vi "Progress Bar Example.vi"() -> ()   [LabVIEW 2015]
uses:
  <vilib>/Utility/sysdir.llb/System Directory Type.ctl
  Library/New Job Status.vi
  Library/New Item Status.vi
  Library/New Item Progression.vi
  Library/Finish.vi
  Library/Simple Progress Bar.lvlib
panel:
  out "Waiting for User":bool
  out "error out":errorcluster
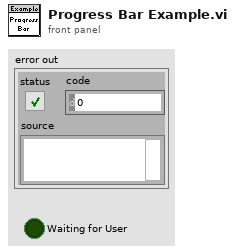
[diagram p1: front panel]
types:
  T1 = typedef "Simple Progress Bar.lvlib/Process Events.ctl" = cluster{"Explorer":refnum<user-event>, "Finished":refnum<user-event>, "Aborted":refnum<user-event>, "New Job":refnum<user-event>, "Item Status":refnum<user-event>, "Item Progression":refnum<user-event>, "Error":refnum<user-event>}
  T2 = typedef "System Directory Type.ctl" = i32
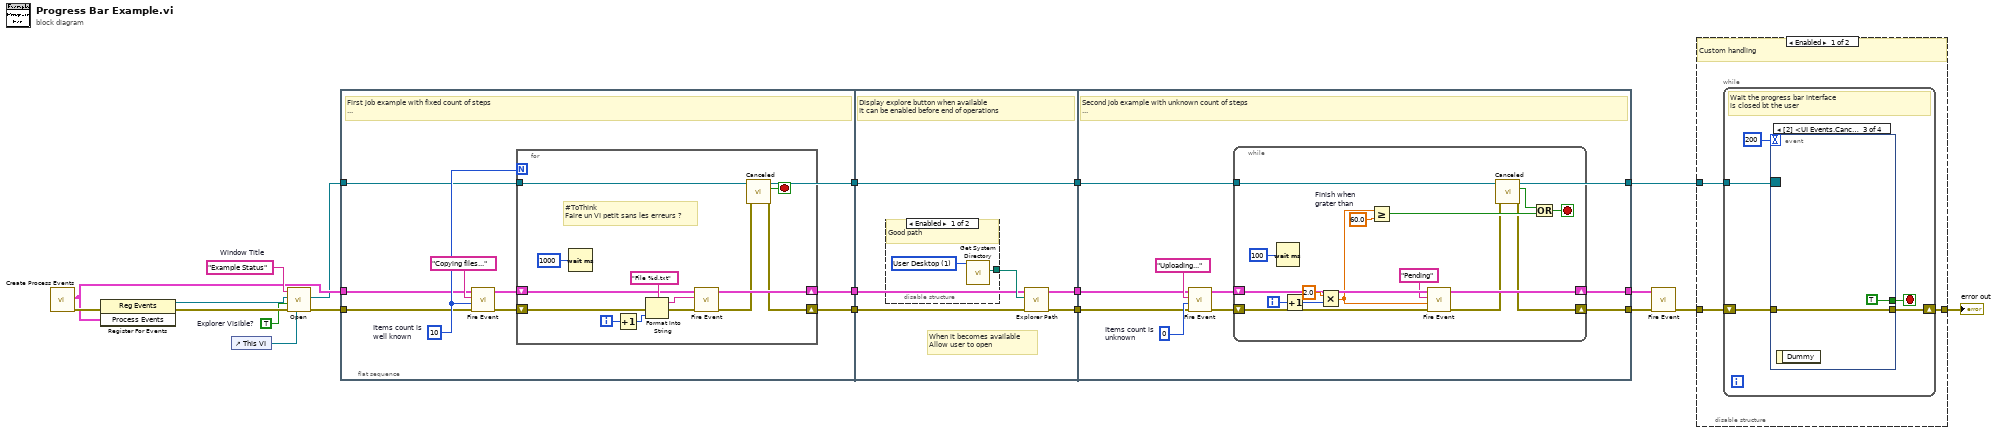
[diagram p0: block diagram]
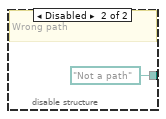
[diagram p2: hidden frame]
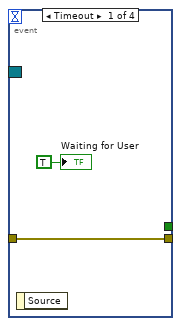
[diagram p3: hidden frame]
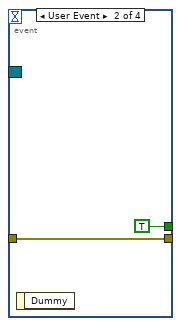
[diagram p4: hidden frame]
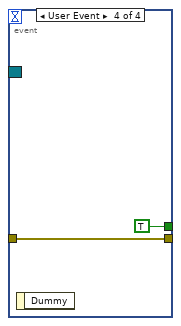
[diagram p5: hidden frame]
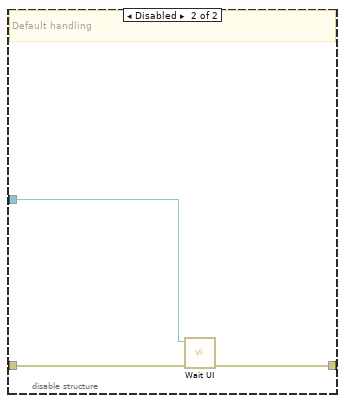
[diagram p6: hidden frame]
diagram:
  w14 = "Example Status"  # Window Title
  w16 = TRUE  # Explorer Visible?
  n1 = call "Create Process Events.vi"() -> ("error out"=w20:errorcluster, "Process Events"=w13:T1)  [unwired: 10 in]
  n2 = register-events(error in=w20, w13) -> (reference out=w15:refnum<event-registration>, error out=w19:errorcluster)  [unwired: 1 in]
  n3 = control-ref of="This VI"() -> (w1:refnum<vi>)
  n4 = call "Open.vi"("VI"=w1, "error in (no error)"=w19, "Explorer Visible? (F)"=w16, "Process Events Registration"=w15, "Window Title"=w14) -> ("error out"=w12:errorcluster, "UI Events Registration"=w11:refnum<event-registration>)  [unwired: 5 in]
  n5 = flat-sequence {
    tunnel: w13 -> [w23]
    tunnel: w12 -> [w22]
    tunnel: w11 -> [w21]
    tunnel: [w25] -> w10
    tunnel: [w24] -> w9
    tunnel: [w21] -> w6
    tunnel: w10 -> [w47]
    tunnel: w9 -> [w45]
    tunnel: [w46] -> w8
    tunnel: [w44] -> w7
    tunnel: w6 -> [w43]
    tunnel: [w43] -> w5
    tunnel: [w53] -> w3
    tunnel: [w54] -> w4
    tunnel: w8 -> [w56]
    tunnel: w7 -> [w55]
    tunnel: w5 -> [w52]
    tunnel: [w52] -> w2
    frame #0 {
      w27 = 10  # Items count is  well known
      # "First job example with fixed count of steps\n..."
      n6 = call-poly "Fire Event.vi"("error in (no error)"=w22, "Items (unknown)"=w27, "Status"="Copying files...", "Process Events"=w23) -> ("error out"=w28:errorcluster, "Process Events out"=w29:T1)  [unwired: 6 in]
      n7 = for {
        N: w27 -> [_]
        shift-right: [w32] -> w25
        shift-left: w28 -> [w42]
        shift-right: [w35] -> w24
        shift-left: w29 -> [w36]
        tunnel: w21 -> [w30]
        i -> [w41]
        stop <- w31 stop-if-true
        # "#ToThink\nFaire un VI petit sans les erreurs ?"
        n8 = Wait (ms)(milliseconds to wait=u32 1000) -> ()  [unwired: 1 out]
        n9 = Increment(x=w41) -> (x+1=w40:i32)
        n10 = Format Into String(format string="File %d.txt", error in=w42, w40) -> (resulting string=w34:string, error out=w37:errorcluster)  [unwired: 1 in]
        n11 = call-poly "Fire Event.vi"("error in (no error)"=w37, "Status"=w34, "Process Events"=w36) -> ("error out"=w33:errorcluster, "Process Events out"=w35:T1)  [unwired: 7 in]
        n12 = call "Canceled.vi"("error in (no error)"=w33, "UI Events Registration"=w30) -> ("error out"=w32:errorcluster, "Canceled by user?"=w31:bool)  [unwired: 8 in]
      }
    }
    frame #1 {
      # "When it becomes available\nAllow user to open"
      # "Display explore button when available\nIt can be enabled before end of operations"
      n13 = disable-structure shown="Enabled" {
        disable-tunnel: [w49 path "Not a path" ("Explorer Path")] -> w48
        frame Enabled {
          w50 = T2 1 items=["User Home"=0, "User Desktop"=1, "User Documents"=2, "User Application Data"=3, "User Preferences"=4, "User Temporary"=5, "Public Documents"=6, "Public Application Data"=7, "Public Preferences"=8, "Public Cache"=13, "System Core Libraries"=9, "System Installed Libraries"=10, "Application Files"=11, "Boot Volume Root"=12] ("system directory type")
          # "Good path"
          n14 = call <vilib>:"Get System Directory.vi"("system directory type"=w50) -> ("system directory"=w49:path)  [unwired: 10 in]
        }
        frame Disabled {
          # "Wrong path"
        }
      }
      n15 = call "Explorer Path.vi"("error in (no error)"=w47, "Explorer Path"=w48, "Process Events"=w45) -> ("error out"=w46:errorcluster, "Process Events out"=w44:T1)  [unwired: 7 in]
    }
    frame #2 {
      w57 = 0  # Items count is  unknown
      # "Second job example with unknown count of steps\n..."
      n16 = call-poly "Fire Event.vi"("error in (no error)"=w56, "Items (unknown)"=w57, "Status"="Uploading...", "Process Events"=w55) -> ("error out"=w59:errorcluster, "Process Events out"=w60:T1)  [unwired: 6 in]
      n17 = while {
        shift-right: [w64] -> w54
        shift-left: w59 -> [w72]
        shift-right: [w71] -> w53
        shift-left: w60 -> [w70]
        tunnel: w52 -> [w63]
        i -> [w74]
        stop <- w62 stop-if-true
        w67 = 60.0  # Finish when  grater than
        n18 = Wait (ms)(milliseconds to wait=u32 100) -> ()  [unwired: 1 out]
        n19 = Increment(x=w74) -> (x+1=w73:i32)
        n20 = Multiply(x=2.0, y=w73) -> (x*y=w68:dbl)
        n21 = Greater Or Equal?(x=w68, y=w67) -> (x >= y?=w66:bool)
        n22 = call-poly "Fire Event.vi"("error in (no error)"=w72, "Progression"=w68, "Status"="Pending", "Process Events"=w70) -> ("error out"=w65:errorcluster, "Process Events out"=w71:T1)  [unwired: 6 in]
        n23 = call "Canceled.vi"("error in (no error)"=w65, "UI Events Registration"=w63) -> ("error out"=w64:errorcluster, "Canceled by user?"=w61:bool)  [unwired: 8 in]
        n24 = Or(x=w61, y=w66) -> (x .or. y?=w62:bool)
      }
    }
  }
  n25 = call-poly "Fire Event.vi"("error in (no error)"=w4, "Process Events"=w3) -> ("error out"=w17:errorcluster)  [unwired: 8 in, 1 out]
  n26 = disable-structure shown="Enabled" {
    disable-tunnel: [w79 w94] -> w18
    disable-tunnel: w17 -> [w78 w95]
    disable-tunnel: w2 -> [w77 w93]
    frame Enabled {
      # "Custom handling"
      n27 = while {
        shift-right: [w83] -> w79
        shift-left: w78 -> [w84]
        tunnel: w77 -> [w80]
        stop <- w82 stop-if-true
        # "Wait the progress bar interface\nis closed bt the user"
        n28 = event shown="[2] <UI Events.Cancel>: User Event" {
          selector: w80 -> [_ _ _ _]
          dyn-events: _ -> [_ _ _ _]
          timeout: 200 -> [_ _ _ _]
          tunnel: [w86 w88 w89 w91] -> w83
          tunnel: w84 -> [w86 w88 w89 w91]
          tunnel: [_ TRUE TRUE TRUE] -> w82
          event Timeout {
            n29 = event-data() -> ()  [unwired: 1 in, 1 out]
            "Waiting for User" <- TRUE ("Waiting for User")
          }
          event User Event {
            n30 = event-data() -> ()  [unwired: 1 in, 1 out]
          }
          event User Event {
            n31 = event-data() -> ()  [unwired: 1 in, 1 out]
          }
          event User Event {
            n32 = event-data() -> ()  [unwired: 1 in, 1 out]
          }
        }
      }
    }
    frame Disabled {
      # "Default handling"
      n33 = call "Wait UI.vi"("error in (no error)"=w95, "UI Events Registration"=w93) -> ("error out"=w94:errorcluster)  [unwired: 7 in, 2 out]
    }
  }
  "error out" <- w18
